vi "GESTIONE PROFILI.vi"() -> ()   [LabVIEW 2019]
uses:
  controls/STEP.ctl
  controls/Caratteristiche step.ctl
  <vilib>/Utility/miscctls.llb/LVRowAndColumnTypeDef.ctl
  <vilib>/addons/database/NI_Database_API.lvlib
  <vilib>/addons/database/Connection.llb/DB Tools Open Connec (String).vi
panel:
  in  "RIMUOVI STEP":bool
  out "ALIMENTATORE 1":cluster{dbl[], dbl[]}[](graph)
  out "FRENO":cluster{dbl[], dbl[]}[](graph)
  in  "Cluster rampa":T2={"Numero step totali"=1.0, "Tempo step [s]"=1.0, "Freno"={"MARCIA"=FALSE, "Control Type"=enum."Speed [RPM]", "RIF iniziale %"=100.0, "RIF finale %"=100.0}, "ALIMENTATORE 1"={"MARCIA"=FALSE, "RIF V iniziale"=100.0, "RIF V FINALE"=100.0, "RIF F INIZIALE"=100.0, "RIF F finale"=100.0}, "ALIMENTATORE 2"={"MARCIA"=FALSE, "RIF V iniziale"=0.0, "RIF F iniziale"=0.0, "RIF V finale"=0.0, "RIF F finale"=0.0}, "Tipo prova"="[-] TUTTE", "Caratteristiche step"={"Attendi stabilizz."=FALSE, "Acq. fine step?"=FALSE, "Acq. automatiche"=FALSE, "PID FRENO"=FALSE, "PID ALIMENTATORE 1"=FALSE, "PID ALIMENTATORE 2"=FALSE, "CAMBIA PROVA SE EQ. TERMICO"=FALSE}} {"Tempo step [s]" min=0.0 max=1000.0; "Numero step totali" min=0.0 max=1000.0}
  in  "MODIFICA STEP":T3={"Tipo prova"="", "Misura resistenza ?"=FALSE, "Tempo Step[s]"=1.0, "Freno"={"MARCIA"=FALSE, "Control Type"=enum."Speed [RPM]", "RIF %"=1.0}, "ALIMENTATORE 1"={"MARCIA"=FALSE, "RIF V"=1.0, "RIF F"=1.0}, "ALIMENTATORE 2"={"MARCIA"=FALSE, "RIF V"=0.0, "RIF F"=0.0}, "Caratteristiche step"={"Attendi stabilizz."=FALSE, "Acq. fine step?"=FALSE, "Acq. automatiche"=FALSE, "PID FRENO"=FALSE, "PID ALIMENTATORE 1"=FALSE, "PID ALIMENTATORE 2"=FALSE, "CAMBIA PROVA SE EQ. TERMICO"=FALSE}} {"Tempo Step[s]" format="%#.1f"}
  in  "ALIMENTAZIONE":T4(radio)
  in  "tipo step":bool caption="STEP SINGOLO\n\nCREA RAMPA"
  in  "SVUOTA":bool
  in  "carica profilo":bool
  in  "NOME PROFILO":string
  in  "ELIMINA PROFILO":bool
  in  "SALVA PROFILO":bool
  in  "LISTA PROFILI ESISTENTI":string(combo)
  in  "INSERISCI STEP NEL PROFILO":bool
  in  "STEP IN MODIFICA":T5={"MODIFICA STEP"={"Tipo prova"="", "Misura resistenza ?"=FALSE, "Tempo Step[s]"=1.0, "Freno"={"MARCIA"=FALSE, "Control Type"=enum."Speed [RPM]", "RIF %"=1.0}, "ALIMENTATORE 1"={"MARCIA"=FALSE, "RIF V"=1.0, "RIF F"=1.0}, "ALIMENTATORE 2"={"MARCIA"=FALSE, "RIF V"=0.0, "RIF F"=0.0}, "Caratteristiche step"={"Attendi stabilizz."=FALSE, "Acq. fine step?"=FALSE, "Acq. automatiche"=FALSE, "PID FRENO"=FALSE, "PID ALIMENTATORE 1"=FALSE, "PID ALIMENTATORE 2"=FALSE, "CAMBIA PROVA SE EQ. TERMICO"=FALSE}}, "MODIFICA STEP"=FALSE, "ELIMINA STEP"=FALSE} {"MODIFICA STEP"."Tempo Step[s]" format="%#.1f"}
  in  "CARICA STEP":bool
  in  "NUOVO STEP":T3={"Tipo prova"="", "Misura resistenza ?"=FALSE, "Tempo Step[s]"=1.0, "Freno"={"MARCIA"=FALSE, "Control Type"=enum."Speed [RPM]", "RIF %"=1.0}, "ALIMENTATORE 1"={"MARCIA"=FALSE, "RIF V"=1.0, "RIF F"=1.0}, "ALIMENTATORE 2"={"MARCIA"=FALSE, "RIF V"=0.0, "RIF F"=0.0}, "Caratteristiche step"={"Attendi stabilizz."=FALSE, "Acq. fine step?"=FALSE, "Acq. automatiche"=FALSE, "PID FRENO"=FALSE, "PID ALIMENTATORE 1"=FALSE, "PID ALIMENTATORE 2"=FALSE, "CAMBIA PROVA SE EQ. TERMICO"=FALSE}} {"Tempo Step[s]" format="%#.1f"}
  in  "LISTA STEP PROFILO":i32(listbox)
  in  "AGGIORNA LISTA PROFILI":bool
  in  "EXIT":bool
  # "UY"
  # "MARCIA ON"
  # "MARCIA OFF"
  # "MARCIA ON"
  # "MARCIA OFF"
  # "NOTA: CLICCA E TRASCINA PER CAMBIARE POSIZIONE AGLI STEP IN TABELLA"
  # "ATTENDI STABILIZZ.: se la grandezza da regolare è stabile, termina lo step prima di raggiungere il tempo step impostato\nACQ. FINE STEP: al termine di uno step, esegui una acquisizione in tabella\nACQ. AUTOMATICHE: permetti le acquisizioni automatiche durante l'esecuzione dello step\nPID FRENO: abilita il pid del freno per la regolazione del setpoint (Potenza, coppia o rpm) impostato\nPID ALIMENTATORE 1: abilita il pid dell'alimentatore per la regolazione del setpoint (V ed F) impostato\nPID ALIMENTATORE 2: non usato\nTERMINA STEP SE EQ. TERMICO: se durante l'esecuzione dello step si verifica il raggiungimento dell'equilibrio termico, termina lo step e passa al successivo"
  # "CARATTERISTICHE STEP:"
  # "Note: Current control type uses the Torque controller. So, if you select  current you will be saving values in torque mode"
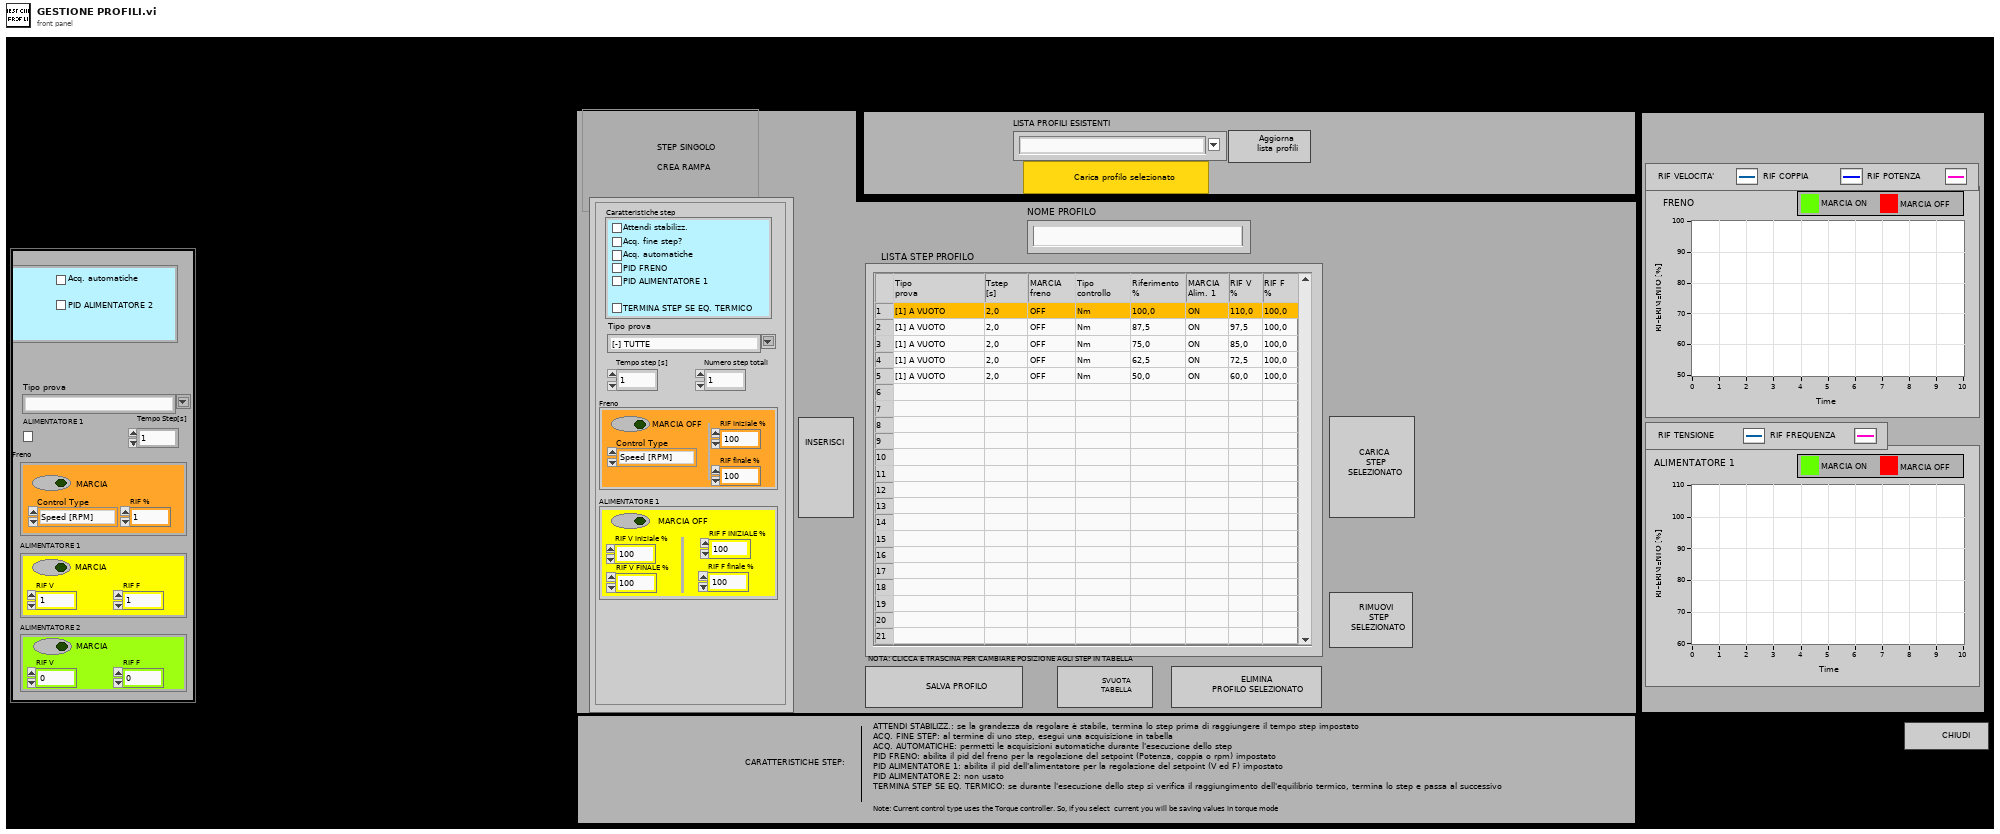
[diagram p1: front panel]
types:
  T1 = typedef "Caratteristiche step.ctl" = cluster{"Attendi stabilizz.":bool, "Acq. fine step?":bool, "Acq. automatiche":bool, "PID FRENO":bool, "PID ALIMENTATORE 1":bool, "PID ALIMENTATORE 2":bool, "CAMBIA PROVA SE EQ. TERMICO":bool}
  T2 = cluster{"Numero step totali":dbl, "Tempo step [s]":dbl, "Freno":cluster{"MARCIA":bool, "Control Type":enum32{"Torque [Nm]", "Power [W]", "Speed [RPM]", "Corrente [A]"}, "RIF iniziale %":dbl, "RIF finale %":dbl}, "ALIMENTATORE 1":cluster{"MARCIA":bool, "RIF V iniziale":dbl, "RIF V FINALE":dbl, "RIF F INIZIALE":dbl, "RIF F finale":dbl}, "ALIMENTATORE 2":cluster{"MARCIA":bool, "RIF V iniziale":dbl, "RIF F iniziale":dbl, "RIF V finale":dbl, "RIF F finale":dbl}, "Tipo prova":string, "Caratteristiche step":T1}
  T3 = typedef "STEP.ctl" = cluster{"Tipo prova":string, "Misura resistenza ?":bool, "Tempo Step[s]":dbl, "Freno":cluster{"MARCIA":bool, "Control Type":enum32{"Torque [Nm]", "Power [W]", "Speed [RPM]", "Corrente [A]"}, "RIF %":dbl}, "ALIMENTATORE 1":cluster{"MARCIA":bool, "RIF V":dbl, "RIF F":dbl}, "ALIMENTATORE 2":cluster{"MARCIA":bool, "RIF V":dbl, "RIF F":dbl}, "Caratteristiche step":T1}
  T4 = enum32{"AC", "DC CON ECCITAZIONE", "DC NO ECCITAZIONE"}
  T5 = cluster{"MODIFICA STEP":T3, "MODIFICA STEP":bool, "ELIMINA STEP":bool}
  T6 = typedef "LVRowAndColumnTypeDef.ctl" = cluster{"Row":i32, "Column":i32}
  T7 = enum16{"open", "replace", "create", "open or create", "replace or create", "replace or create with confirmation"}
  T8 = typedef "NI_Database_API.lvlib/Conn ObjectReference.ctl" = refnum<k1>
  T9 = cluster{"[0]":string, "[1]":string, "[2]":string, "[3]":string, "[4]":string, "[5]":string, "[6]":string, "[7]":string, "[8]":string, "[9]":string, "[10]":string, "[11]":string, "[12]":string, "[13]":string, "[14]":string, "[15]":string, "[16]":string, "[17]":string, "[18]":string, "[19]":string, "[20]":string}
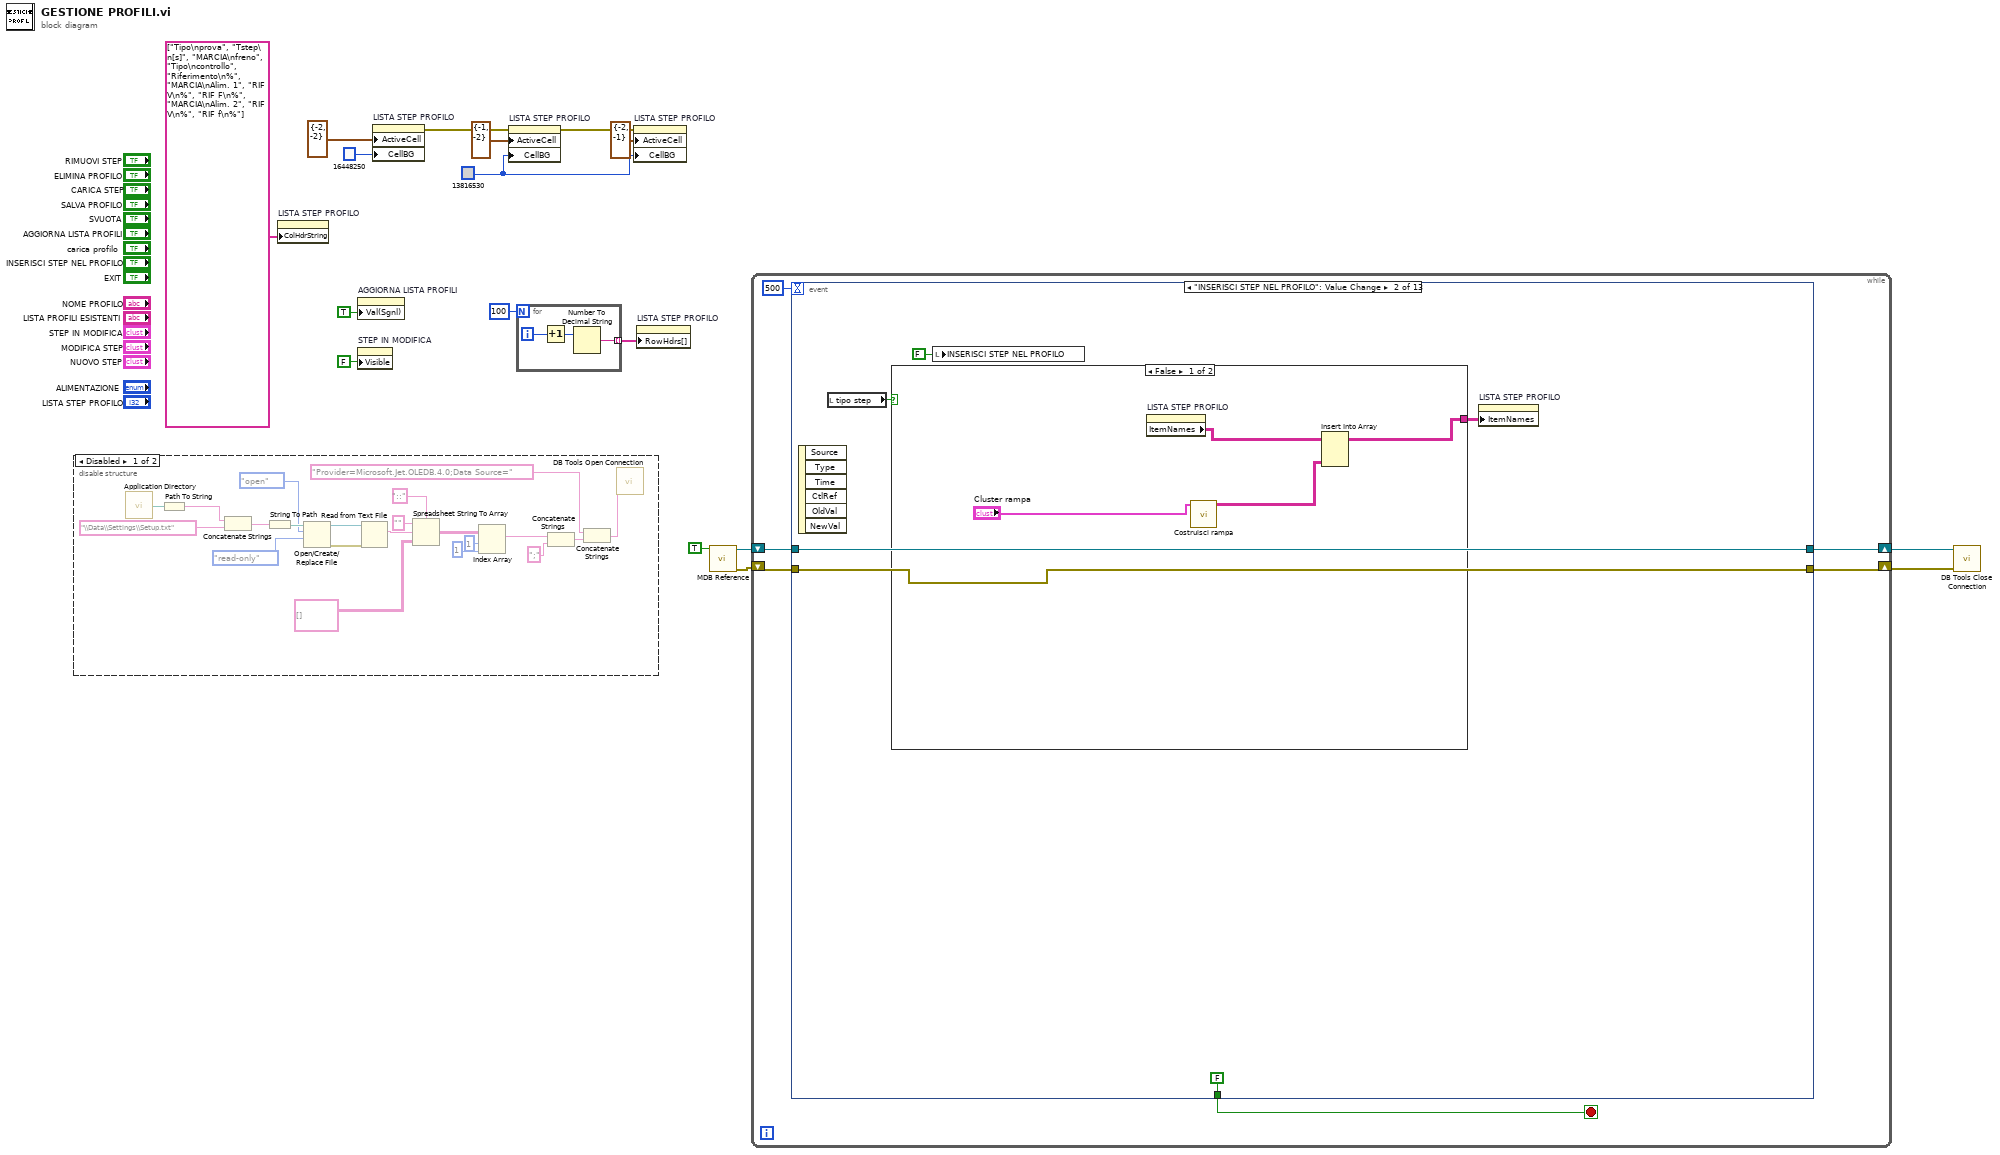
[diagram p0: block diagram]
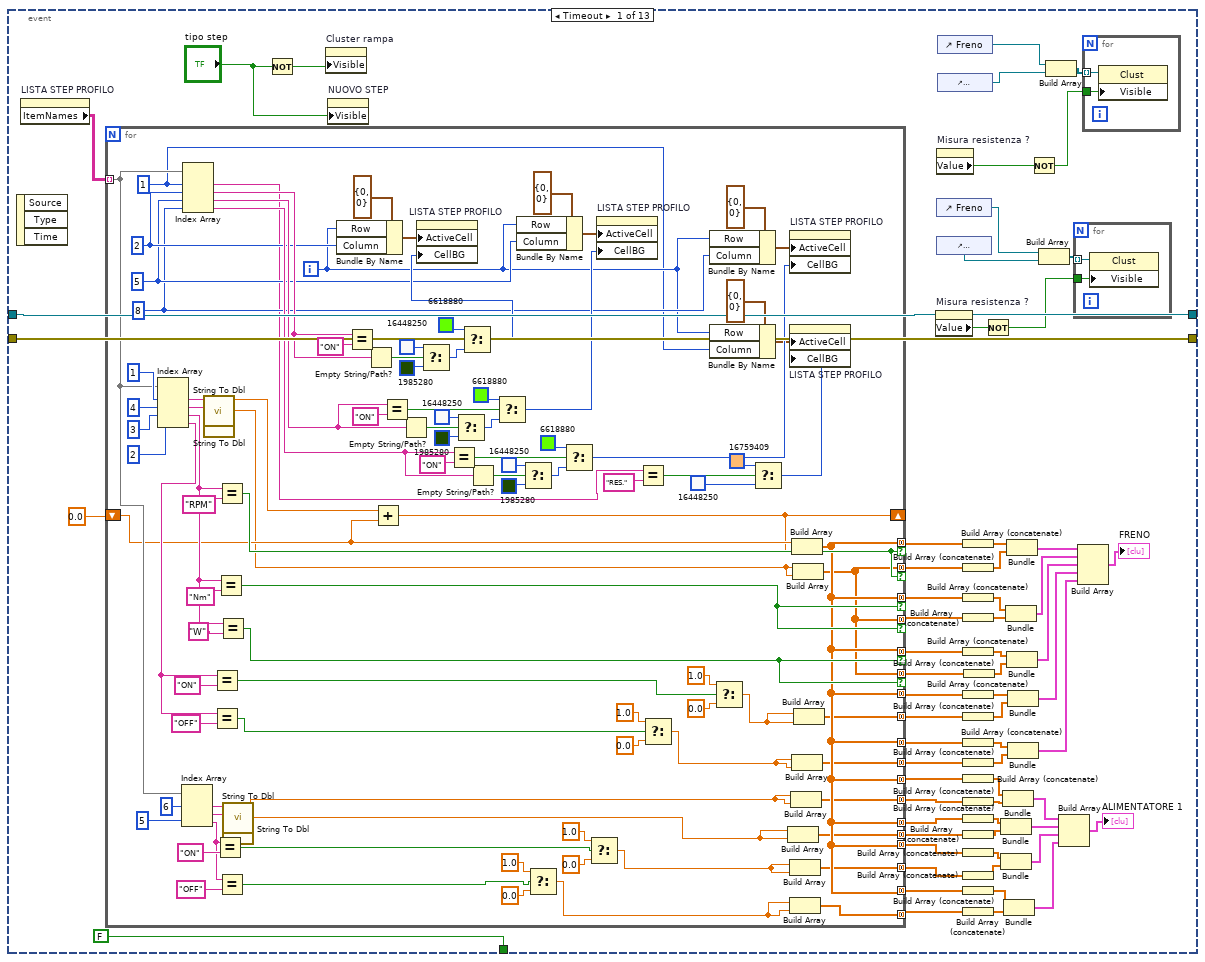
[diagram p3: hidden frame]
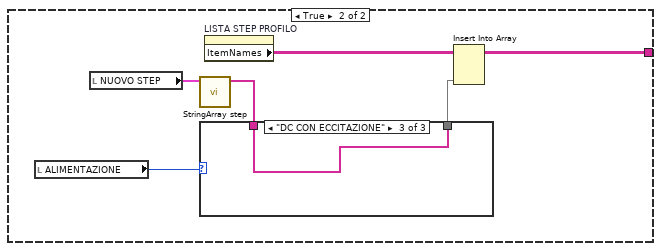
[diagram p4: hidden frame]
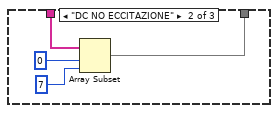
[diagram p6: hidden frame]
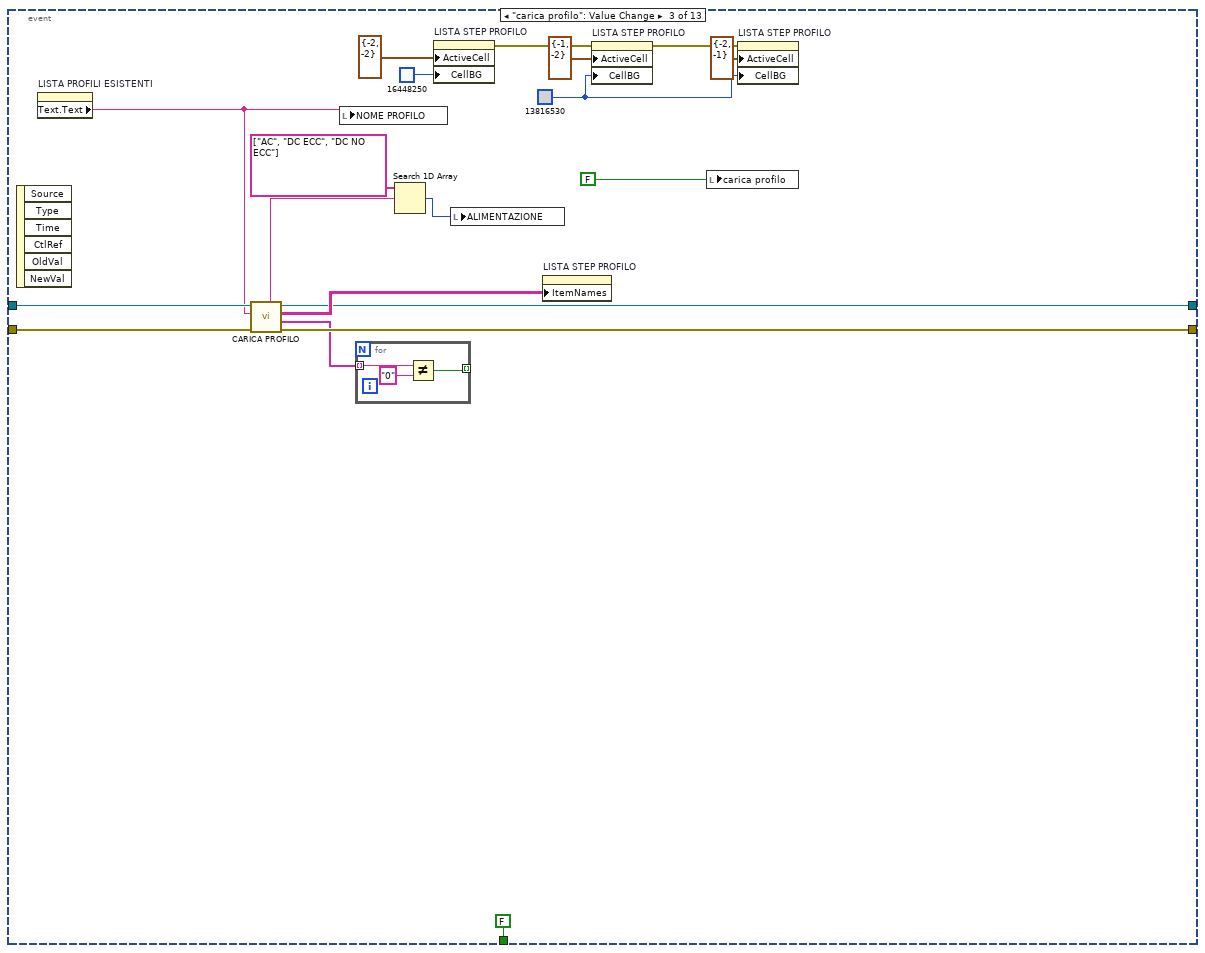
[diagram p7: hidden frame]
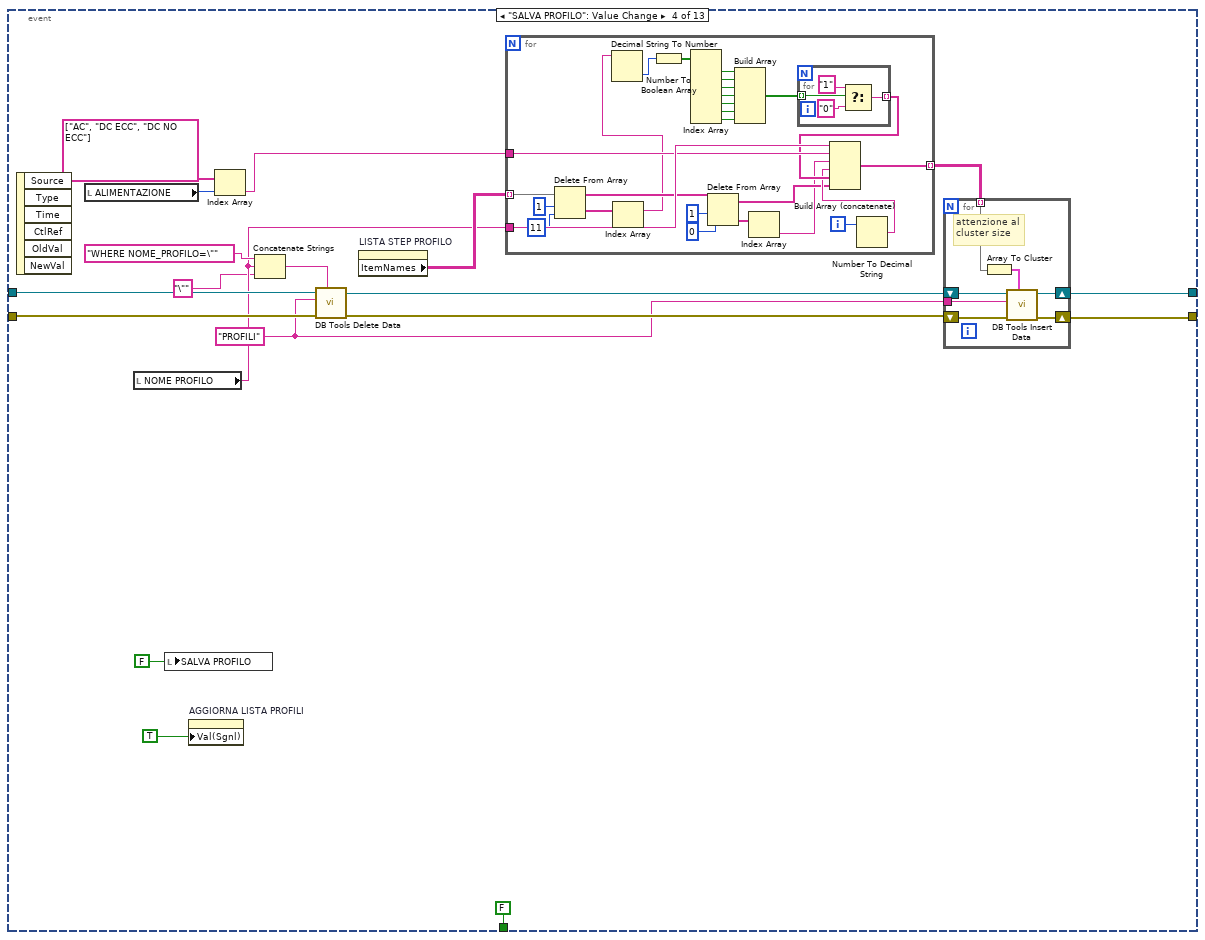
[diagram p8: hidden frame]
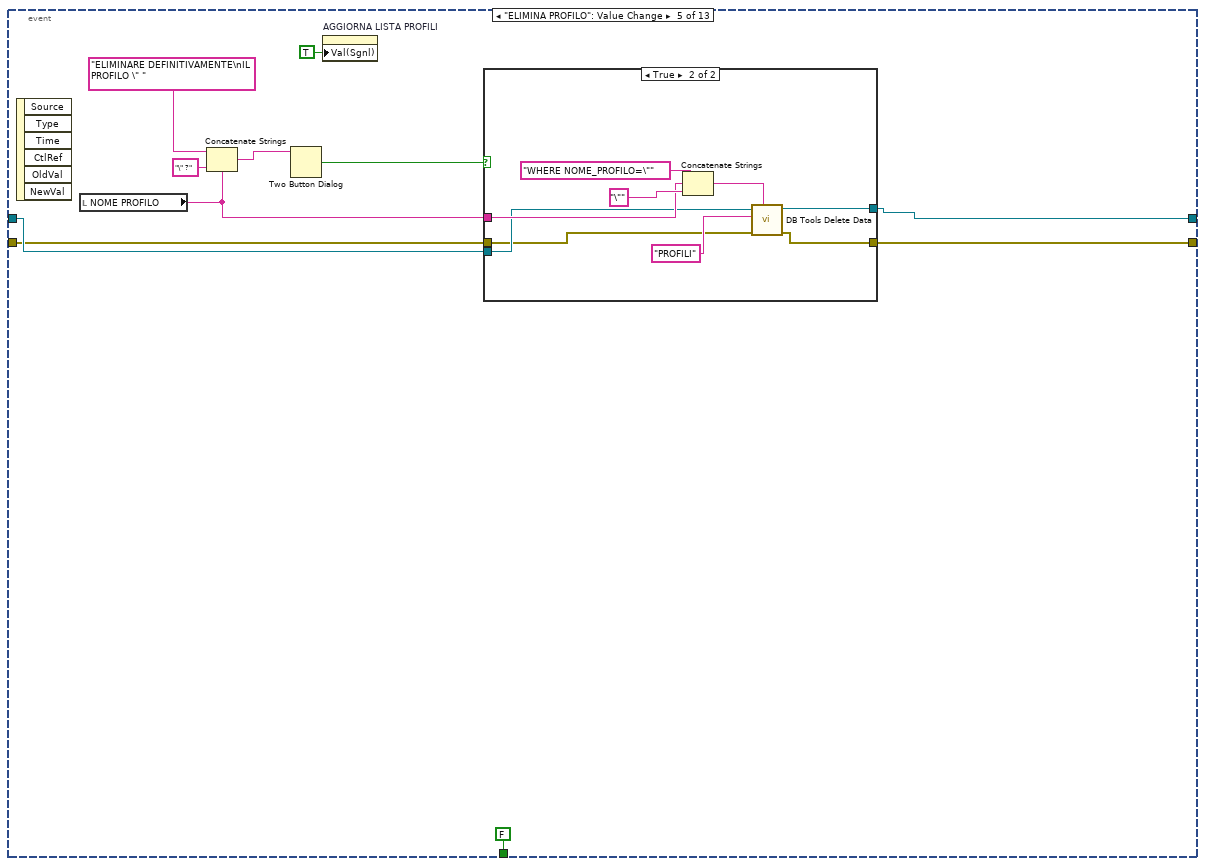
[diagram p9: hidden frame]
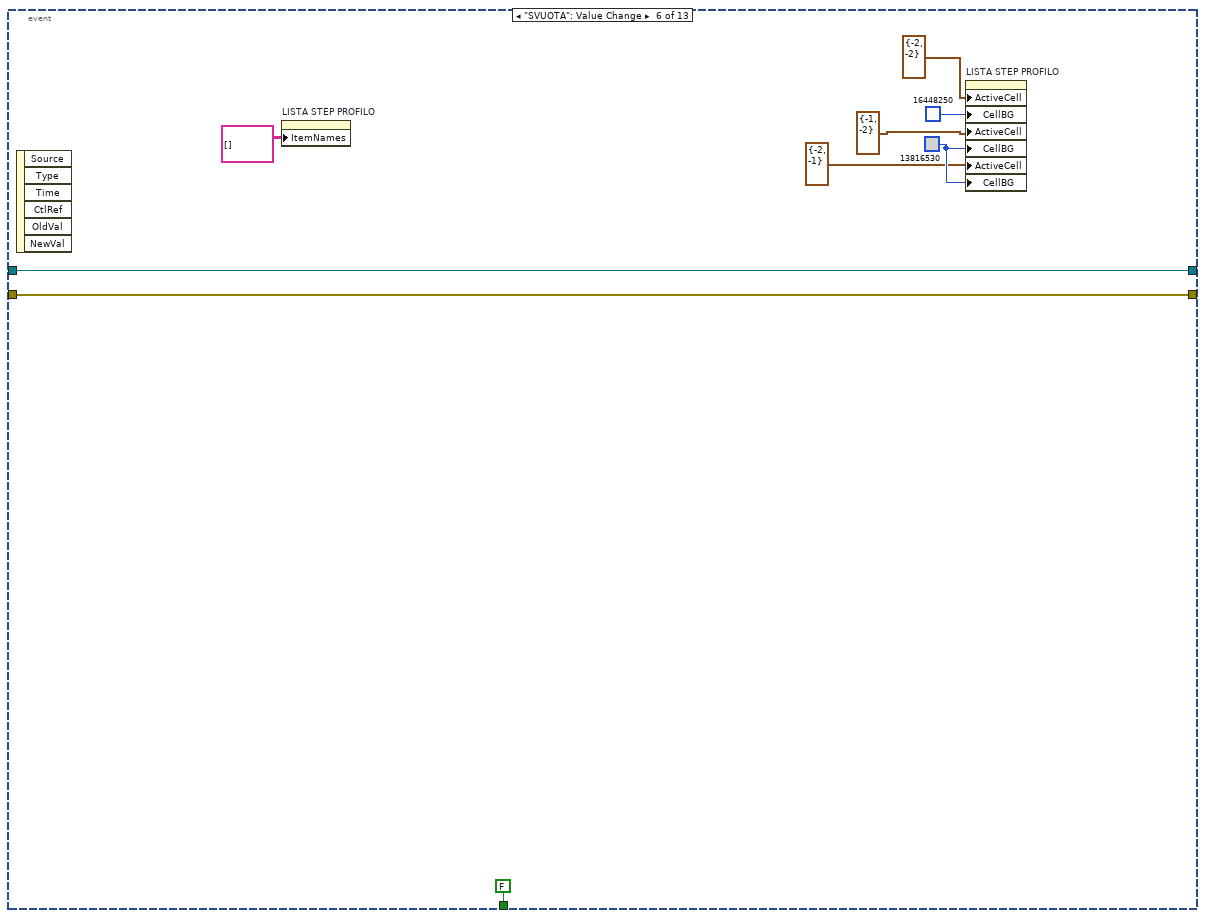
[diagram p11: hidden frame]
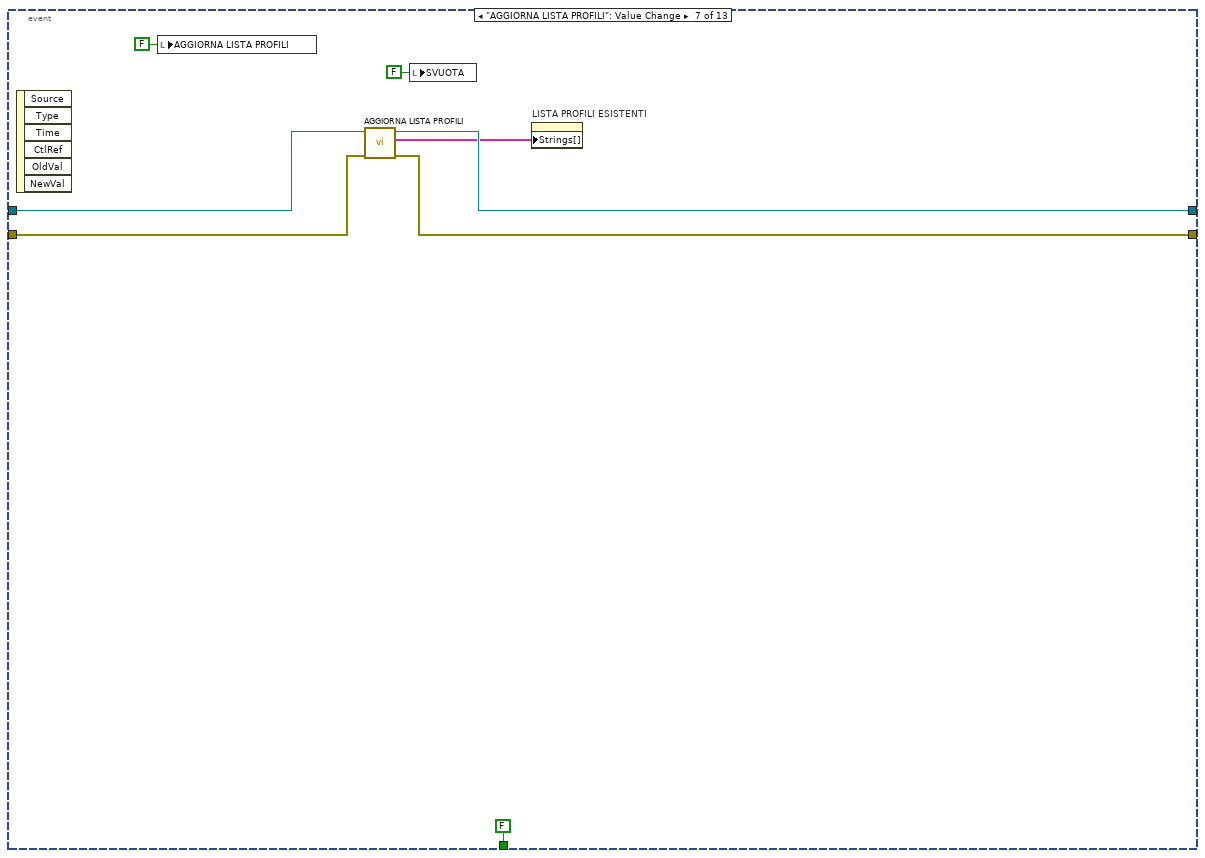
[diagram p12: hidden frame]
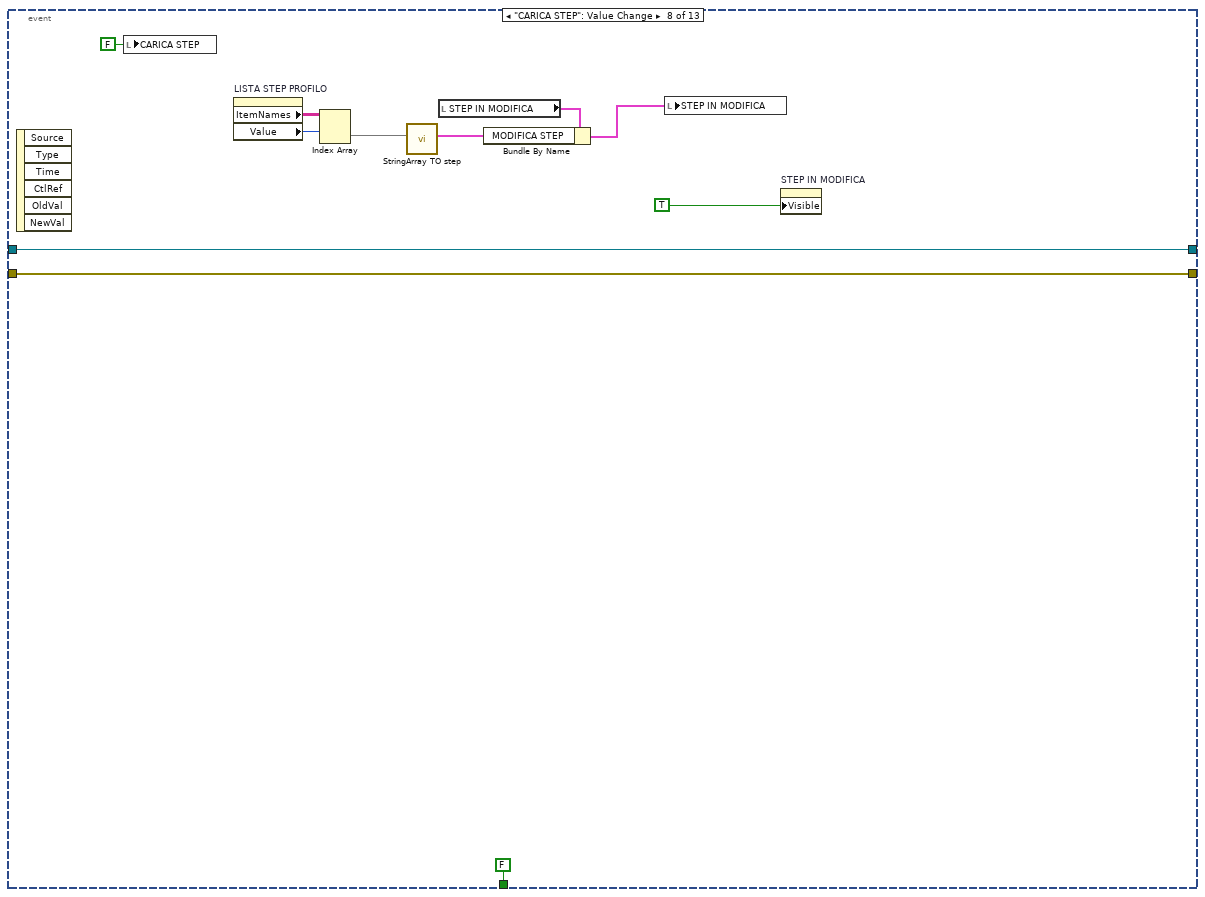
[diagram p13: hidden frame]
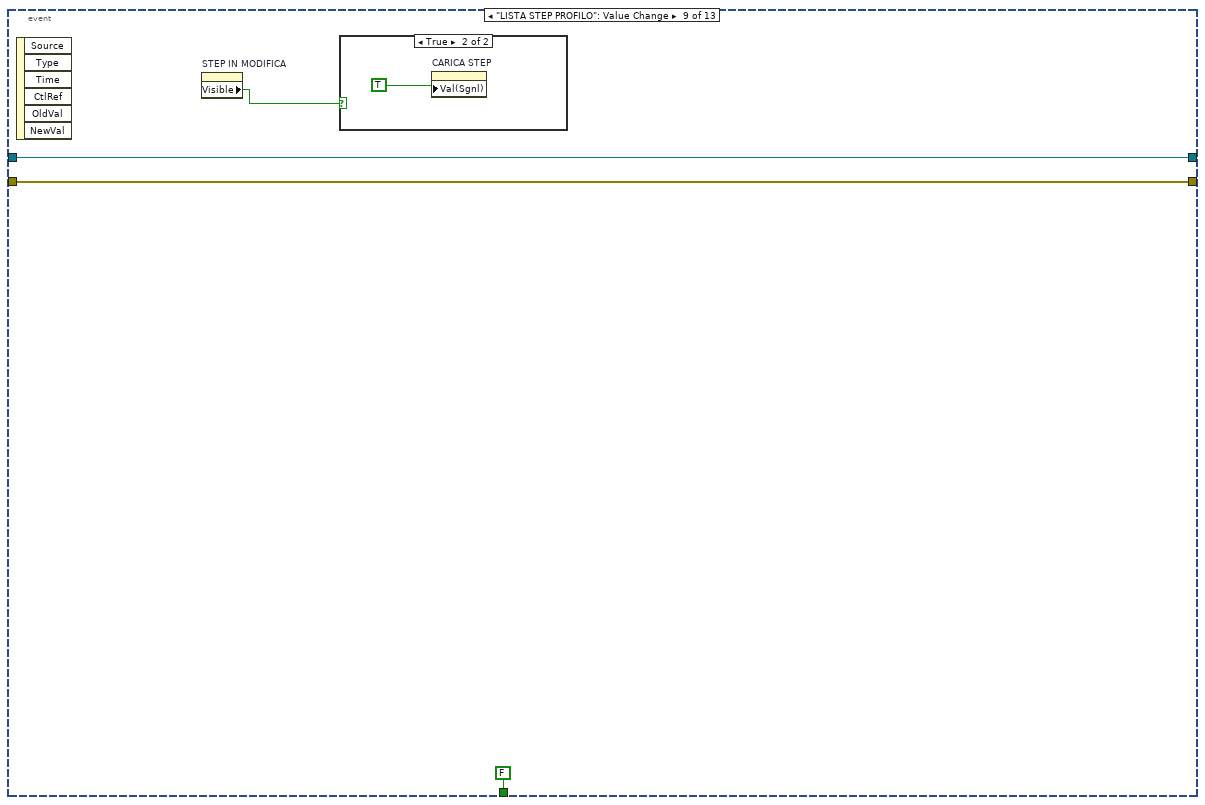
[diagram p14: hidden frame]
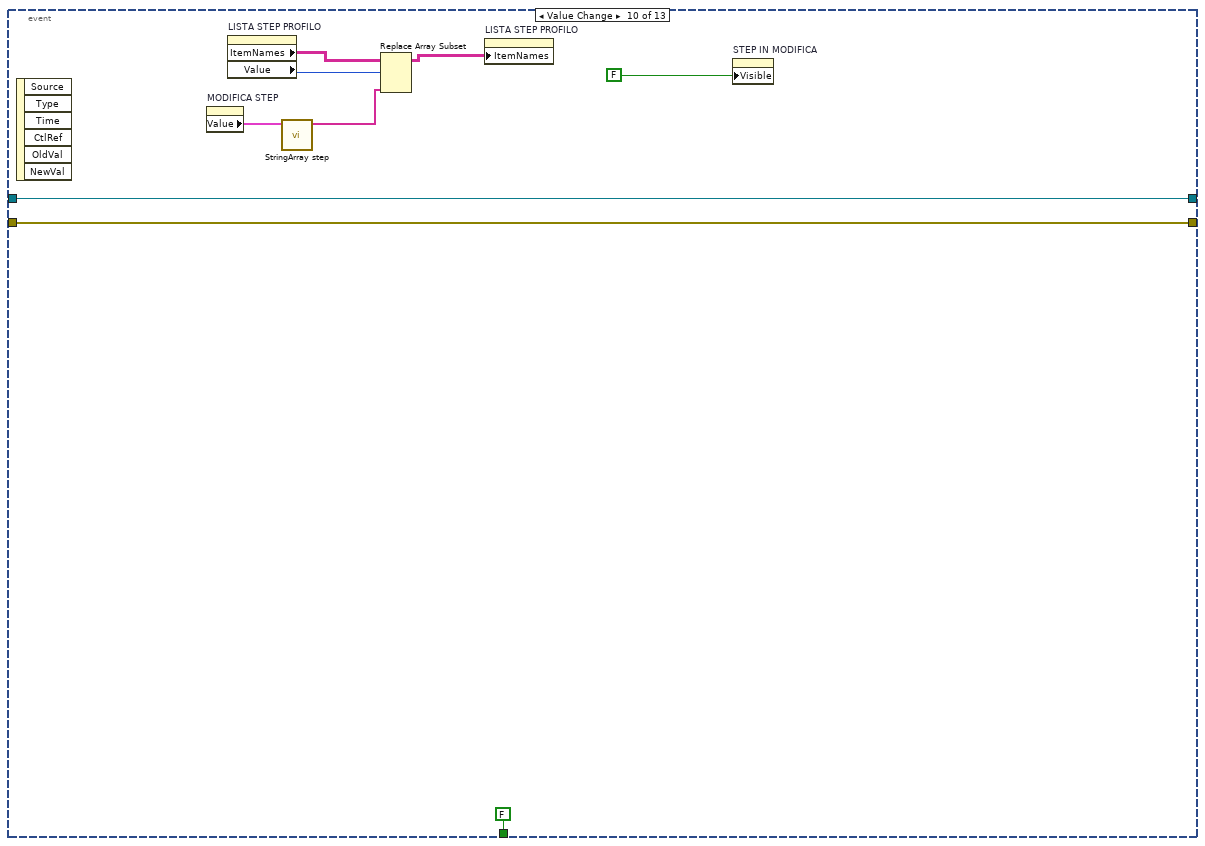
[diagram p16: hidden frame]
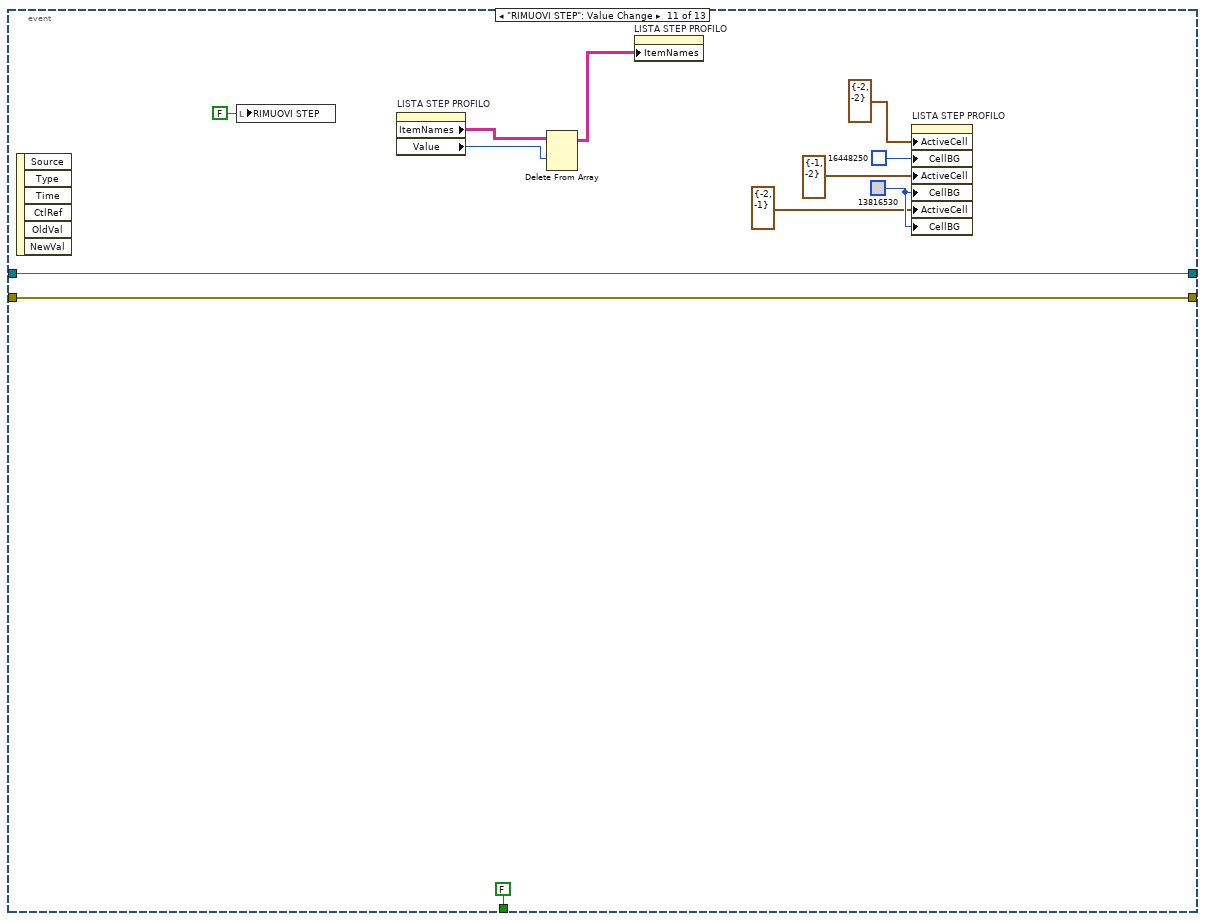
[diagram p17: hidden frame]
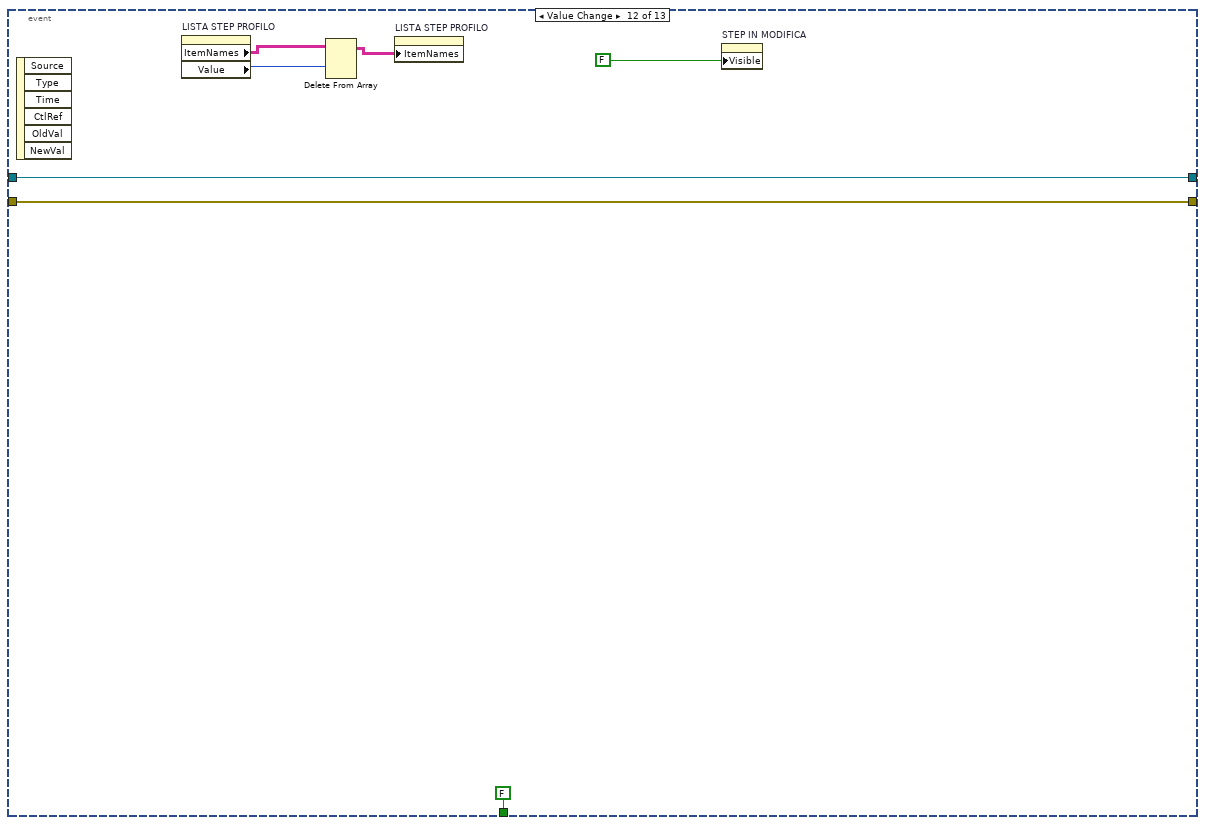
[diagram p18: hidden frame]
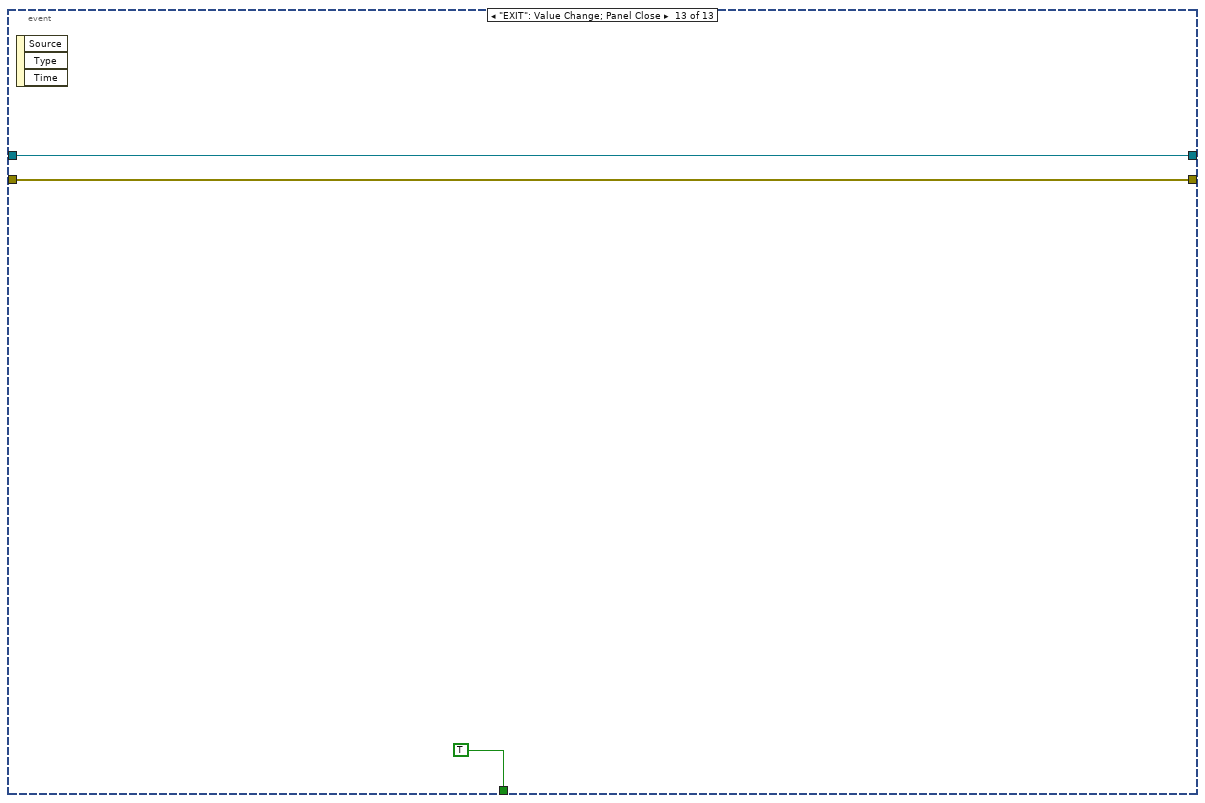
[diagram p19: hidden frame]
diagram:
  w8 = u32 13816530
  n1 = disable-structure shown="Disabled" {
    frame Disabled {
      n2 = call <vilib>:"Application Directory.vi"() -> ("Application Directory"=w26:path)
      n3 = Path To String(path=w26) -> (string=w25:string)
      n4 = Concatenate Strings(w25, "\\Data\\Settings\\Setup.txt" ("string")) -> (w37:string)
      n5 = String To Path(string=w37) -> (path=w35:path)
      n6 = Open/Create/Replace File(file path (use dialog)=w35, operation (0:open)=T7."open", access (0:read/write)=enum16{"read/write", "read-only", "write-only"}."read-only") -> (refnum out=w32:refnum<file>, error out=w31:errorcluster)  [unwired: 3 in, 1 out]
      n7 = Read from Text File(file (use dialog)=w32, error in=w31) -> (text=w30:string)  [unwired: 2 in, 3 out]
      n8 = Spreadsheet String To Array(delimiter (Tab)="::", format string="", spreadsheet string=w30, array type (2D Dbl)=string[][] []) -> (array=w27:string[][])
      n9 = Index Array(array=w27, index (row)=1 ("disabled index (row)"), index (col)=1 ("disabled index (col)")) -> (element=w19:string)
      n10 = Concatenate Strings(w19, ";" ("string")) -> (w20:string)
      n11 = Concatenate Strings("Provider=Microsoft.Jet.OLEDB.4.0;Data Source=" ("string"), w20) -> (w21:string)
      n12 = call-poly <vilib>:"DB Tools Open Connection.vi"("connection information"=w21) -> ()  [unwired: 7 in, 2 out]
    }
    frame Enabled {
    }
  }
  n13 = property on="LISTA STEP PROFILO" class="MCListbox (strict)"("ColHdrString"=string[] ["Tipo\nprova", "Tstep\n[s]", "MARCIA\nfreno", "Tipo\ncontrollo", "Riferimento\n%", "MARCIA\nAlim. 1", "RIF V\n%", "RIF F\n%", "MARCIA\nAlim. 2", "RIF V\n%", "RIF f\n%"] ("Column Header Strings[]")) -> ()  [unwired: 2 in, 2 out]
  n14 = property on="AGGIORNA LISTA PROFILI" class="Bool (strict)"("Val(Sgnl)"=TRUE ("Value (Signaling)")) -> ()  [unwired: 2 in, 2 out]
  n15 = property on="STEP IN MODIFICA" class="Clust (strict)"("Visible"=FALSE) -> ()  [unwired: 2 in, 2 out]
  n16 = property on="LISTA STEP PROFILO" class="MCListbox (strict)"("ActiveCell"=T6 {"Row"=-2, "Column"=-2} ("Active Cell:Active Cell"), "CellBG"=u32 16448250) -> (error out=w4:errorcluster)  [unwired: 2 in, 1 out]
  n17 = property on="LISTA STEP PROFILO" class="MCListbox (strict)"(error in=w4, "ActiveCell"=T6 {"Row"=-1, "Column"=-2} ("Active Cell:Active Cell"), "CellBG"=w8) -> (error out=w6:errorcluster)  [unwired: 1 in, 1 out]
  n18 = for {
    N: 100 -> [_]
    tunnel: [w39] -> w13 mode=indexing
    i -> [w41]
    n19 = Increment(x=w41) -> (x+1=w40:i32)
    n20 = Number To Decimal String(number=w40) -> (decimal integer string=w39:string)  [unwired: 1 in]
  }
  n21 = property on="LISTA STEP PROFILO" class="MCListbox (strict)"(error in=w6, "ActiveCell"=T6 {"Row"=-2, "Column"=-1} ("Active Cell:Active Cell"), "CellBG"=w8) -> ()  [unwired: 1 in, 2 out]
  n22 = property on="LISTA STEP PROFILO" class="MCListbox (strict)"("RowHdrs[]"=w13) -> ()  [unwired: 2 in, 2 out]
  n23 = call "MDB Reference.vi"("Collaudi T/motori F"=TRUE) -> ("error out"=w9:errorcluster, "Refnum out"=w10:T8)  [unwired: 8 in, 1 out]
  n24 = while {
    shift-right: [w46] -> w17
    shift-left: w10 -> [w47]
    shift-right: [w44] -> w16
    shift-left: w9 -> [w45]
    stop <- w43 stop-if-true
    n25 = event shown="[1] \"INSERISCI STEP NEL PROFILO\": Value Change" {
      selector: _ -> [_ _ _ _ _ _ _ _ _ _ _ _ _]
      dyn-events: _ -> [_ _ _ _ _ _ _ _ _ _ _ _ _]
      timeout: 500 -> [_ _ _ _ _ _ _ _ _ _ _ _ _]
      tunnel: w47 -> [w111 w220 w256 w277 w322 w346 w355 w363 w369 w380 w388 w395 w401]
      tunnel: [w111 w220 w252 w267 w320 w346 w354 w363 w369 w380 w388 w395 w401] -> w46
      tunnel: w45 -> [w110 w219 w255 w276 w321 w345 w353 w362 w368 w379 w387 w394 w400]
      tunnel: [w110 w219 w251 w266 w319 w345 w352 w362 w368 w379 w387 w394 w400] -> w44
      tunnel: [FALSE FALSE FALSE FALSE FALSE FALSE FALSE FALSE FALSE FALSE FALSE FALSE TRUE] -> w43
      event Timeout {
        n26 = event-data() -> ()  [unwired: 1 in, 3 out]
        n27 = property on="LISTA STEP PROFILO" class="MCListbox (strict)"() -> ("ItemNames"=w108:string[][])  [unwired: 2 in, 2 out]
        n28 = for {
          tunnel: w108 -> [w167] mode=indexing
          shift-right: [w143] -> _
          shift-left: 0.0 -> [w157]
          tunnel: [w144] -> w105 mode=concatenating if=w175
          tunnel: [w142] -> w104 mode=concatenating if=w175
          tunnel: [w144] -> w101 mode=concatenating if=w173
          tunnel: [w142] -> w100 mode=concatenating if=w173
          tunnel: [w144] -> w98 mode=concatenating if=w170
          tunnel: [w142] -> w97 mode=concatenating if=w170
          tunnel: [w144] -> w95 mode=concatenating
          tunnel: [w139] -> w94 mode=concatenating
          tunnel: [w144] -> w92 mode=concatenating
          tunnel: [w135] -> w91 mode=concatenating
          tunnel: [w144] -> w90 mode=concatenating
          tunnel: [w133] -> w89 mode=concatenating
          tunnel: [w144] -> w88 mode=concatenating
          tunnel: [w131] -> w87 mode=concatenating
          tunnel: [w144] -> w85 mode=concatenating
          tunnel: [w137] -> w84 mode=concatenating
          tunnel: [w144] -> w82 mode=concatenating
          tunnel: [w129] -> w81 mode=concatenating
          i -> [w117]
          w116 = 1 ("index")
          w126 = 8 ("index")
          w127 = 5 ("index")
          w128 = 2 ("Column")
          n29 = Index Array(array=w167, index #1=1 ("index"), index #2=4 ("index"), index #3=3 ("index"), index #4=2 ("index")) -> (element #1=w180:string, element #2=w179:string, element #3=w171:string, element #4=w160:string)
          n30 = Index Array(array=w167, index #1=6 ("index"), index #3=5 ("index")) -> (element #1=w164:string, element #2=w163:string, element #3=w158:string)  [unwired: 1 in]
          n31 = Index Array(array=w167, index #1=w116, index #2=w128, index #3=w127, index #4=w126) -> (element #1=w120:string, element #2=w184:string, element #3=w193:string, element #4=w202:string)
          n32 = call "String To Dbl.vi"("String"=w180) -> ("Numeric"=w178:dbl)  [unwired: 10 in]
          n33 = call "String To Dbl.vi"("String"=w179) -> ("Numeric"=w141:dbl)  [unwired: 10 in]
          n34 = Equal?(x=w160, y="ON") -> (x = y?=w156:bool)
          n35 = Equal?(x=w160, y="OFF") -> (x = y?=w152:bool)
          n36 = Equal?(x=w158, y="ON") -> (x = y?=w148:bool)
          n37 = Equal?(x=w171, y="Nm") -> (x = y?=w173:bool)
          n38 = Equal?(x=w171, y="RPM") -> (x = y?=w175:bool)
          n39 = Equal?(x=w158, y="OFF") -> (x = y?=w145:bool)
          n40 = Equal?(x=w171, y="W") -> (x = y?=w170:bool)
          n41 = call "String To Dbl.vi"("String"=w164) -> ("Numeric"=w136:dbl)  [unwired: 10 in]
          n42 = call "String To Dbl.vi"("String"=w163) -> ("Numeric"=w134:dbl)  [unwired: 10 in]
          n43 = Bundle By Name(cluster=T6 {"Row"=0, "Column"=0} ("Active Cell:Active Cell"), "Row"=w117, "Column"=w128) -> (w214:T6)
          n44 = Equal?(x=w184, y="ON") -> (x = y?=w189:bool)
          n45 = Empty String/Path?(string/path=w184) -> (empty?=w186:bool)
          n46 = Add(x=w178, y=w157) -> (x+y=w143:dbl)
          n47 = Equal?(x=w193, y="ON") -> (x = y?=w196:bool)
          n48 = Empty String/Path?(string/path=w193) -> (empty?=w199:bool)
          n49 = Select(t=u32 16448250, s=w186, f=u32 1985280) -> (s? t:f=w187:u32)
          n50 = Equal?(x=w202, y="ON") -> (x = y?=w207:bool)
          n51 = Select(t=u32 16448250, s=w199, f=u32 1985280) -> (s? t:f=w198:u32)
          n52 = Select(t=u32 6618880, s=w189, f=w187) -> (s? t:f=w183:u32)
          n53 = property on="LISTA STEP PROFILO" class="MCListbox (strict)"("ActiveCell"=w214, "CellBG"=w183) -> ()  [unwired: 2 in, 2 out]
          n54 = Empty String/Path?(string/path=w202) -> (empty?=w203:bool)
          n55 = Select(t=u32 6618880, s=w196, f=w198) -> (s? t:f=w192:u32)
          n56 = Bundle By Name(cluster=T6 {"Row"=0, "Column"=0} ("Active Cell:Active Cell"), "Row"=w117, "Column"=w127) -> (w213:T6)
          n57 = Select(t=u32 16448250, s=w203, f=u32 1985280) -> (s? t:f=w204:u32)
          n58 = Select(t=1.0, s=w145, f=0.0) -> (s? t:f=w130:dbl)
          n59 = Select(t=u32 6618880, s=w207, f=w204) -> (s? t:f=w206:u32)
          n60 = Select(t=1.0, s=w148, f=0.0) -> (s? t:f=w132:dbl)
          n61 = property on="LISTA STEP PROFILO" class="MCListbox (strict)"("ActiveCell"=w213, "CellBG"=w192) -> ()  [unwired: 2 in, 2 out]
          n62 = Equal?(x=w120, y="RES.") -> (x = y?=w123:bool)
          n63 = Select(t=1.0, s=w152, f=0.0) -> (s? t:f=w138:dbl)
          n64 = Bundle By Name(cluster=T6 {"Row"=0, "Column"=0} ("Active Cell:Active Cell"), "Row"=w117, "Column"=w126) -> (w210:T6)
          n65 = Bundle By Name(cluster=T6 {"Row"=0, "Column"=0} ("Active Cell:Active Cell"), "Row"=w117, "Column"=w116) -> (w125:T6)
          n66 = Select(t=1.0, s=w156, f=0.0) -> (s? t:f=w140:dbl)
          n67 = Select(t=u32 16759409, s=w123, f=u32 16448250) -> (s? t:f=w118:u32)
          n68 = Build Array(w134, w134) -> (w133:dbl[])
          n69 = property on="LISTA STEP PROFILO" class="MCListbox (strict)"("ActiveCell"=w210, "CellBG"=w206) -> ()  [unwired: 2 in, 2 out]
          n70 = property on="LISTA STEP PROFILO" class="MCListbox (strict)"("ActiveCell"=w125, "CellBG"=w118) -> ()  [unwired: 2 in, 2 out]
          n71 = Build Array(w132, w132) -> (w131:dbl[])
          n72 = Build Array(w130, w130) -> (w129:dbl[])
          n73 = Build Array(w136, w136) -> (w135:dbl[])
          n74 = Build Array(w157, w143) -> (w144:dbl[])
          n75 = Build Array(w138, w138) -> (w137:dbl[])
          n76 = Build Array(w141, w141) -> (w142:dbl[])
          n77 = Build Array(w140, w140) -> (w139:dbl[])
        }
        n78 = Not(x="tipo step") -> (.not. x?=w107:bool)
        n79 = property on="Cluster rampa" class="Clust (strict)"("Visible"=w107) -> ()  [unwired: 2 in, 2 out]
        n80 = property on="NUOVO STEP" class="Clust (strict)"("Visible"="tipo step") -> ()  [unwired: 2 in, 2 out]
        n81 = property on="Misura resistenza ?" class="Bool (strict)"() -> ("Value"=w54:bool)  [unwired: 2 in, 2 out]
        n82 = property on="Misura resistenza ?" class="Bool (strict)"() -> ("Value"=w58:bool)  [unwired: 2 in, 2 out]
        n83 = control-ref of="Freno"() -> (w51:refnum<vi>)
        n84 = control-ref of="ALIMENTATORE 1"() -> (w52:refnum<vi>)
        n85 = control-ref of="Freno"() -> (w55:refnum<vi>)
        n86 = control-ref of="ALIMENTATORE 1"() -> (w56:refnum<vi>)
        n87 = Build Array (concatenate)(w105) -> (w80:dbl[])
        n88 = Build Array (concatenate)(w104) -> (w79:dbl[])
        n89 = Build Array (concatenate)(w101) -> (w78:dbl[])
        n90 = Build Array (concatenate)(w100) -> (w77:dbl[])
        n91 = Build Array (concatenate)(w98) -> (w76:dbl[])
        n92 = Build Array (concatenate)(w95) -> (w74:dbl[])
        n93 = Build Array (concatenate)(w94) -> (w73:dbl[])
        n94 = Build Array (concatenate)(w85) -> (w72:dbl[])
        n95 = Build Array (concatenate)(w84) -> (w71:dbl[])
        n96 = Build Array (concatenate)(w92) -> (w70:dbl[])
        n97 = Build Array (concatenate)(w91) -> (w69:dbl[])
        n98 = Build Array (concatenate)(w90) -> (w68:dbl[])
        n99 = Build Array (concatenate)(w89) -> (w67:dbl[])
        n100 = Build Array (concatenate)(w88) -> (w66:dbl[])
        n101 = Build Array (concatenate)(w87) -> (w65:dbl[])
        n102 = Build Array (concatenate)(w82) -> (w64:dbl[])
        n103 = Build Array (concatenate)(w81) -> (w63:dbl[])
        n104 = Build Array (concatenate)(w97) -> (w75:dbl[])
        n105 = Not(x=w54) -> (.not. x?=w49:bool)
        n106 = Bundle(w68, w67) -> (w61:cluster{dbl[], dbl[]})  [unwired: 1 in]
        n107 = Bundle(w66, w65) -> (w60:cluster{dbl[], dbl[]})  [unwired: 1 in]
        n108 = Bundle(w70, w69) -> (w86:cluster{dbl[], dbl[]})  [unwired: 1 in]
        n109 = Bundle(w64, w63) -> (w59:cluster{dbl[], dbl[]})  [unwired: 1 in]
        n110 = Bundle(w78, w77) -> (w99:cluster{dbl[], dbl[]})  [unwired: 1 in]
        n111 = Bundle(w80, w79) -> (w103:cluster{dbl[], dbl[]})  [unwired: 1 in]
        n112 = Bundle(w76, w75) -> (w96:cluster{dbl[], dbl[]})  [unwired: 1 in]
        n113 = Bundle(w74, w73) -> (w93:cluster{dbl[], dbl[]})  [unwired: 1 in]
        n114 = Bundle(w72, w71) -> (w83:cluster{dbl[], dbl[]})  [unwired: 1 in]
        n115 = Not(x=w58) -> (.not. x?=w50:bool)
        n116 = Build Array(w51, w52) -> (w53:refnum<vi>[])
        n117 = Build Array(w55, w56) -> (w57:refnum<vi>[])
        n118 = Build Array(w86, w61, w60, w59) -> (→"ALIMENTATORE 1":cluster{dbl[], dbl[]}[])
        n119 = for {
          tunnel: w53 -> [w113] mode=indexing
          tunnel: w49 -> [w112]
          n120 = property class="Clust"(reference=w113, "Visible"=w112) -> ()  [unwired: 1 in, 2 out]
        }
        n121 = Build Array(w103, w99, w96, w93, w83) -> (→"FRENO":cluster{dbl[], dbl[]}[])
        n122 = for {
          tunnel: w57 -> [w115] mode=indexing
          tunnel: w50 -> [w114]
          n123 = property class="Clust"(reference=w115, "Visible"=w114) -> ()  [unwired: 1 in, 2 out]
        }
      }
      event "INSERISCI STEP NEL PROFILO": Value Change {
        n124 = event-data() -> ()  [unwired: 1 in, 6 out]
        n125 = local read "tipo step"() -> (w217:bool)
        n126 = case shown="False" w217 {
          tunnel: [w224 w230] -> w221
          frame False {
            n127 = property on="LISTA STEP PROFILO" class="MCListbox (strict)"() -> ("ItemNames"=w225:string[][])  [unwired: 2 in, 2 out]
            n128 = call "Costruisci rampa.vi"("Cluster rampa"="Cluster rampa") -> ("Array"=w222:string[][])  [unwired: 10 in]
            n129 = Insert Into Array "Insert Into Array"(array=w225, new element=w222) -> (w224:string[][])  [unwired: 2 in]
          }
          frame True {
            n130 = local read "ALIMENTAZIONE"() -> (w226:T4)
            n131 = local read "NUOVO STEP"() -> (w229:T3)
            n132 = call "StringArray step.vi"("NUOVO STEP"=w229) -> ("Array"=w228:string[])  [unwired: 10 in]
            n133 = case shown="\"DC CON ECCITAZIONE\"" w226 {
              tunnel: w228 -> [w232 w236 w237]
              tunnel: [w232 w235 w237] -> w227
              frame "AC", Default {
              }
              frame "DC NO ECCITAZIONE" {
                n134 = Array Subset(array=w236, index=0, length=7) -> (w235:string[])
              }
              frame "DC CON ECCITAZIONE" {
              }
            }
            n135 = property on="LISTA STEP PROFILO" class="MCListbox (strict)"() -> ("ItemNames"=w231:string[][])  [unwired: 2 in, 2 out]
            n136 = Insert Into Array(array=w231, new element=w227) -> (w230:string[][])  [unwired: 2 in]
          }
        }
        n137 = local write "INSERISCI STEP NEL PROFILO"(FALSE ("INSERISCI STEP NEL PROFILO")) -> ()
        n138 = property on="LISTA STEP PROFILO" class="MCListbox (strict)"("ItemNames"=w221) -> ()  [unwired: 2 in, 2 out]
      }
      event "carica profilo": Value Change {
        w239 = u32 13816530
        n139 = event-data() -> ()  [unwired: 1 in, 6 out]
        n140 = property on="LISTA PROFILI ESISTENTI" class="CmbBox"() -> ("Text.Text"=w253:string)  [unwired: 2 in, 2 out]
        n141 = call "CARICA PROFILO.vi"("error in (no error)"=w255, "Text.Text"=w253, "Refnum in"=w256) -> ("error out"=w251:errorcluster, "Array"=w249:string[], "Step profilo"=w254:string[][], "Refnum out"=w252:T8, "tipo collegamento"=w247:string)  [unwired: 3 in, 1 out]
        n142 = local write "NOME PROFILO"(w253) -> ()
        n143 = for {
          tunnel: w249 -> [w259] mode=indexing
          tunnel: [w257] -> _ mode=indexing
          n144 = Not Equal?(x=w259, y="0") -> (x != y?=w257:bool)
        }
        n145 = Search 1D Array(1D array=string[] ["AC", "DC ECC", "DC NO ECC"], element=w247) -> (index of element=w246:i32)  [unwired: 1 in]
        n146 = property on="LISTA STEP PROFILO" class="MCListbox (strict)"("ActiveCell"=T6 {"Row"=-2, "Column"=-2} ("Active Cell:Active Cell"), "CellBG"=u32 16448250) -> (error out=w243:errorcluster)  [unwired: 2 in, 1 out]
        n147 = local write "ALIMENTAZIONE"(w246) -> ()
        n148 = property on="LISTA STEP PROFILO" class="MCListbox (strict)"("ItemNames"=w254) -> ()  [unwired: 2 in, 2 out]
        n149 = property on="LISTA STEP PROFILO" class="MCListbox (strict)"(error in=w243, "ActiveCell"=T6 {"Row"=-1, "Column"=-2} ("Active Cell:Active Cell"), "CellBG"=w239) -> (error out=w241:errorcluster)  [unwired: 1 in, 1 out]
        n150 = local write "carica profilo"(FALSE ("carica profilo")) -> ()
        n151 = property on="LISTA STEP PROFILO" class="MCListbox (strict)"(error in=w241, "ActiveCell"=T6 {"Row"=-2, "Column"=-1} ("Active Cell:Active Cell"), "CellBG"=w239) -> ()  [unwired: 1 in, 2 out]
      }
      event "SALVA PROFILO": Value Change {
        w269 = "PROFILI" ("table")
        n152 = event-data() -> ()  [unwired: 1 in, 6 out]
        n153 = local read "ALIMENTAZIONE"() -> (w262:T4)
        n154 = local read "NOME PROFILO"() -> (w273:string)
        n155 = local write "SALVA PROFILO"(FALSE ("SALVA PROFILO")) -> ()
        n156 = property on="AGGIORNA LISTA PROFILI" class="Bool (strict)"("Val(Sgnl)"=TRUE ("Value (Signaling)")) -> ()  [unwired: 2 in, 2 out]
        n157 = Index Array(array=string[] ["AC", "DC ECC", "DC NO ECC"], index=w262) -> (element=w261:string)
        n158 = Concatenate Strings("WHERE NOME_PROFILO=\"" ("condition"), w273, "\"" ("string")) -> (w274:string)
        n159 = call <vilib>:"DB Tools Delete Data.vi"("condition"=w274, "error in (no error)"=w276, "table"=w269, "connection reference"=w277) -> ("error out"=w271:errorcluster, "connection reference out"=w270:T8)  [unwired: 6 in]
        n160 = property on="LISTA STEP PROFILO" class="MCListbox (strict)"() -> ("ItemNames"=w278:string[][])  [unwired: 2 in, 2 out]
        n161 = for {
          tunnel: w278 -> [w294] mode=indexing
          tunnel: [w312] -> w268 mode=indexing
          tunnel: w273 -> [w310]
          tunnel: w261 -> [w309]
          i -> [w311]
          n162 = Delete From Array(array=w294, length=1, index=11) -> (deleted portion=w298:string[], array with subset deleted=w287:string[])
          n163 = Index Array(array=w298) -> (element=w286:string)  [unwired: 1 in]
          n164 = Decimal String To Number(string=w286) -> (number=w307:i32)  [unwired: 2 in, 1 out]
          n165 = Number To Boolean Array(number=w307) -> (Boolean array=w299:bool[])
          n166 = Index Array(array=w299) -> (element #1=w300:bool, element #2=w301:bool, element #3=w302:bool, element #4=w303:bool, element #5=w304:bool, element #6=w305:bool, element #7=w306:bool)  [unwired: 7 in]
          n167 = Delete From Array(array=w287, length=1, index=0) -> (deleted portion=w290:string[], array with subset deleted=w291:string[])
          n168 = Build Array(w300, w301, w302, w303, w304, w305, w306) -> (w297:bool[])
          n169 = Index Array(array=w290) -> (element=w289:string)  [unwired: 1 in]
          n170 = for {
            tunnel: w297 -> [w316] mode=indexing
            tunnel: [w313] -> w296 mode=indexing
            n171 = Select(t="1", s=w316, f="0") -> (s? t:f=w313:string)
          }
          n172 = Number To Decimal String(number=w311) -> (decimal integer string=w295:string)  [unwired: 1 in]
          n173 = Build Array (concatenate)(w310, w309, w289, w295, w296, w291) -> (w312:string[])
        }
        n174 = for {
          tunnel: w269 -> [w283]
          tunnel: w268 -> [w282] mode=indexing
          shift-right: [w280] -> w266
          shift-left: w271 -> [w285]
          shift-right: [w281] -> w267
          shift-left: w270 -> [w284]
          # "attenzione al\ncluster size"
          n175 = Array To Cluster(array=w282) -> (cluster=w279:T9)
          n176 = call <vilib>:"DB Tools Insert Data.vi"("data"=w279, "error in (no error)"=w285, "table"=w283, "connection reference"=w284) -> ("error out"=w280:errorcluster, "connection reference out"=w281:T8)  [unwired: 6 in]
        }
      }
      event "ELIMINA PROFILO": Value Change {
        n177 = event-data() -> ()  [unwired: 1 in, 6 out]
        n178 = local read "NOME PROFILO"() -> (w323:string)
        n179 = Concatenate Strings("ELIMINARE DEFINITIVAMENTE\nIL PROFILO \" " ("message"), w323, "\" ?" ("string")) -> (w326:string)
        n180 = Two Button Dialog(message=w326) -> (T button?=w324:bool)  [unwired: 2 in]
        n181 = property on="AGGIORNA LISTA PROFILI" class="Bool (strict)"("Val(Sgnl)"=TRUE ("Value (Signaling)")) -> ()  [unwired: 2 in, 2 out]
        n182 = case shown="True" w324 {
          tunnel: w323 -> [_ w334]
          tunnel: w322 -> [w329 w333]
          tunnel: w321 -> [w328 w332]
          tunnel: [w329 w331] -> w320
          tunnel: [w328 w330] -> w319
          frame False {
          }
          frame True {
            n183 = Concatenate Strings("WHERE NOME_PROFILO=\"" ("condition"), w334, "\"" ("string")) -> (w337:string)
            n184 = call <vilib>:"DB Tools Delete Data.vi"("condition"=w337, "error in (no error)"=w332, "table"="PROFILI", "connection reference"=w333) -> ("error out"=w330:errorcluster, "connection reference out"=w331:T8)  [unwired: 6 in]
          }
        }
      }
      event "SVUOTA": Value Change {
        w341 = u32 13816530
        n185 = event-data() -> ()  [unwired: 1 in, 6 out]
        n186 = property on="LISTA STEP PROFILO" class="MCListbox (strict)"("ItemNames"=string[][] [] ("Item Names")) -> ()  [unwired: 2 in, 2 out]
        n187 = property on="LISTA STEP PROFILO" class="MCListbox (strict)"("ActiveCell"=T6 {"Row"=-2, "Column"=-2} ("Active Cell:Active Cell"), "CellBG"=u32 16448250, "ActiveCell"=T6 {"Row"=-1, "Column"=-2} ("Active Cell:Active Cell"), "CellBG"=w341, "ActiveCell"=T6 {"Row"=-2, "Column"=-1} ("Active Cell:Active Cell"), "CellBG"=w341) -> ()  [unwired: 2 in, 2 out]
      }
      event "AGGIORNA LISTA PROFILI": Value Change {
        n188 = event-data() -> ()  [unwired: 1 in, 6 out]
        n189 = local write "AGGIORNA LISTA PROFILI"(FALSE ("AGGIORNA LISTA PROFILI")) -> ()
        n190 = call "AGGIORNA LISTA PROFILI.vi"("error in (no error)"=w353, "Refnum in"=w355) -> ("error out"=w352:errorcluster, "Array"=w351:string[], "Refnum out"=w354:T8)  [unwired: 7 in]
        n191 = local write "SVUOTA"(FALSE ("SVUOTA")) -> ()
        n192 = property on="LISTA PROFILI ESISTENTI" class="CmbBox"("Strings[]"=w351) -> ()  [unwired: 2 in, 2 out]
      }
      event "CARICA STEP": Value Change {
        n193 = event-data() -> ()  [unwired: 1 in, 6 out]
        n194 = local write "CARICA STEP"(FALSE ("CARICA STEP")) -> ()
        n195 = property on="LISTA STEP PROFILO" class="MCListbox (strict)"() -> ("ItemNames"=w366:string[][], "Value"=w365:i32)  [unwired: 2 in, 2 out]
        n196 = Index Array(array=w366, index (row)=w365) -> (element=w364:string[])  [unwired: 1 in]
        n197 = call "StringArray TO step.vi"("ItemNames"=w364) -> ("STEP"=w357:T3)  [unwired: 10 in]
        n198 = local read "STEP IN MODIFICA"() -> (w359:T5)
        n199 = Bundle By Name(cluster=w359, "MODIFICA STEP"=w357) -> (w358:T5)
        n200 = local write "STEP IN MODIFICA"(w358) -> ()
        n201 = property on="STEP IN MODIFICA" class="Clust (strict)"("Visible"=TRUE) -> ()  [unwired: 2 in, 2 out]
      }
      event "LISTA STEP PROFILO": Value Change {
        n202 = event-data() -> ()  [unwired: 1 in, 6 out]
        n203 = property on="STEP IN MODIFICA" class="Clust (strict)"() -> ("Visible"=w370:bool)  [unwired: 2 in, 2 out]
        n204 = case shown="True" w370 {
          frame False {
          }
          frame True {
            n205 = property on="CARICA STEP" class="Bool (strict)"("Val(Sgnl)"=TRUE) -> ()  [unwired: 2 in, 2 out]
          }
        }
      }
      event "STEP IN MODIFICA.MODIFICA STEP": Value Change {
        n206 = event-data() -> ()  [unwired: 1 in, 6 out]
        n207 = property on="MODIFICA STEP" class="Clust (strict)"() -> ("Value"=w374:T3)  [unwired: 2 in, 2 out]
        n208 = property on="LISTA STEP PROFILO" class="MCListbox (strict)"() -> ("ItemNames"=w378:string[][], "Value"=w377:i32)  [unwired: 2 in, 2 out]
        n209 = call "StringArray step.vi"("NUOVO STEP"=w374) -> ("Array"=w373:string[])  [unwired: 10 in]
        n210 = Replace Array Subset(array=w378, new element=w373, index (row)=w377) -> (w376:string[][])  [unwired: 1 in]
        n211 = property on="LISTA STEP PROFILO" class="MCListbox (strict)"("ItemNames"=w376) -> ()  [unwired: 2 in, 2 out]
        n212 = property on="STEP IN MODIFICA" class="Clust (strict)"("Visible"=FALSE) -> ()  [unwired: 2 in, 2 out]
      }
      event "RIMUOVI STEP": Value Change {
        w383 = u32 13816530
        n213 = event-data() -> ()  [unwired: 1 in, 6 out]
        n214 = local write "RIMUOVI STEP"(FALSE ("RIMUOVI STEP")) -> ()
        n215 = property on="LISTA STEP PROFILO" class="MCListbox (strict)"() -> ("ItemNames"=w391:string[][], "Value"=w389:i32)  [unwired: 2 in, 2 out]
        n216 = Delete From Array(array=w391, index (row)=w389) -> (array with subset deleted=w390:string[][])  [unwired: 2 in, 1 out]
        n217 = property on="LISTA STEP PROFILO" class="MCListbox (strict)"("ItemNames"=w390) -> ()  [unwired: 2 in, 2 out]
        n218 = property on="LISTA STEP PROFILO" class="MCListbox (strict)"("ActiveCell"=T6 {"Row"=-2, "Column"=-2} ("Active Cell:Active Cell"), "CellBG"=u32 16448250, "ActiveCell"=T6 {"Row"=-1, "Column"=-2} ("Active Cell:Active Cell"), "CellBG"=w383, "ActiveCell"=T6 {"Row"=-2, "Column"=-1} ("Active Cell:Active Cell"), "CellBG"=w383) -> ()  [unwired: 2 in, 2 out]
      }
      event "STEP IN MODIFICA.ELIMINA STEP": Value Change {
        n219 = event-data() -> ()  [unwired: 1 in, 6 out]
        n220 = property on="LISTA STEP PROFILO" class="MCListbox (strict)"() -> ("ItemNames"=w399:string[][], "Value"=w398:i32)  [unwired: 2 in, 2 out]
        n221 = Delete From Array(array=w399, index (row)=w398) -> (array with subset deleted=w397:string[][])  [unwired: 2 in, 1 out]
        n222 = property on="LISTA STEP PROFILO" class="MCListbox (strict)"("ItemNames"=w397) -> ()  [unwired: 2 in, 2 out]
        n223 = property on="STEP IN MODIFICA" class="Clust (strict)"("Visible"=FALSE) -> ()  [unwired: 2 in, 2 out]
      }
      event "EXIT": Value Change; Panel Close {
        n224 = event-data() -> ()  [unwired: 1 in, 3 out]
      }
    }
  }
  n225 = call <vilib>:"DB Tools Close Connection.vi"("error in (no error)"=w16, "connection reference"=w17) -> ()  [unwired: 5 in, 1 out]
